vi "Load Outputs.vi"(8 "error in (no error)":errorcluster, 11 "DiscreteRangeControl in":refnum<class "DiscreteRangeControl.lvclass">) -> (0 "error out":errorcluster, 3 "DiscreteRangeControl out":refnum<class "DiscreteRangeControl.lvclass">)   [LabVIEW 2020, in "VolatusControl.lvlib" / "DiscreteRangeControl.lvclass"]
uses:
  DiscreteRangeControl.lvclass
  DiscreteRangeControl.lvclass/DiscreteRangeControl.ctl
  lv-cdm/CDM-Config/Config Element/Config Element.lvclass
  Volatus/MessageQ/MessageQ.lvclass
  Control Action.ctl
  VolatusControl.lvlib
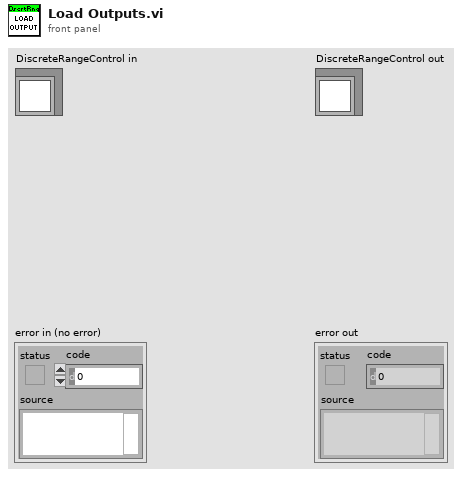
[diagram p1: front panel]
types:
  T1 = typedef "VolatusControl.lvlib/Control Action.ctl" = cluster{"Channel":string, "MsgQ":refnum<class "MessageQ.lvclass">, "Value":bool}
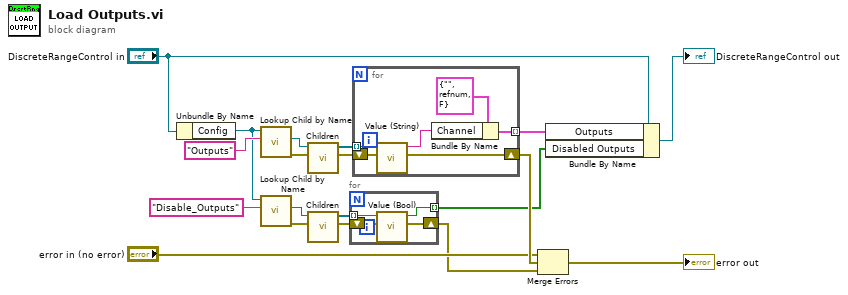
[diagram p0: block diagram]
diagram:
  n1 = Unbundle By Name("DiscreteRangeControl in") -> ("Config"=w9:refnum<class "Config Element.lvclass">)
  n2 = call "Lookup Child by Name.vi"("Name"="Outputs", "Config Element in"=w9) -> ("error out"=w15:errorcluster, "Child"=w14:refnum<class "Config Element.lvclass">)  [unwired: 6 in, 2 out]
  n3 = call "Lookup Child by Name.vi"("Name"="Disable_Outputs", "Config Element in"=w9) -> ("error out"=w6:errorcluster, "Child"=w7:refnum<class "Config Element.lvclass">)  [unwired: 6 in, 2 out]
  n4 = call "Children.vi"("error in (no error)"=w15, "Config Element in"=w14) -> ("error out"=w12:errorcluster, "Elements"=w13:refnum<class "Config Element.lvclass">[])  [unwired: 8 in]
  n5 = call "Children.vi"("error in (no error)"=w6, "Config Element in"=w7) -> ("error out"=w5:errorcluster, "Elements"=w4:refnum<class "Config Element.lvclass">[])  [unwired: 8 in]
  n6 = for {
    shift-right: [w21] -> w1
    shift-left: w5 -> [w23]
    tunnel: w4 -> [w22] mode=indexing
    tunnel: [w20] -> w3 mode=indexing
    n7 = call "Value (Bool).vi"("error in (no error)"=w23, "Config Element in"=w22) -> ("error out"=w21:errorcluster, "Bool Value"=w20:bool)  [unwired: 8 in]
  }
  n8 = for {
    tunnel: w13 -> [w29] mode=indexing
    shift-right: [w24] -> w19
    shift-left: w12 -> [w28]
    tunnel: [w25] -> w10 mode=indexing
    n9 = call "Value (String).vi"("error in (no error)"=w28, "Config Element in"=w29) -> ("error out"=w24:errorcluster, "String Value"=w26:string)  [unwired: 8 in]
    n10 = Bundle By Name(cluster=T1 {"Channel"="", "MsgQ"=refnum, "Value"=FALSE} ("Action"), "Channel"=w26) -> (w25:T1)
  }
  n11 = Merge Errors("error in (no error)", w19, w1) -> (→"error out":errorcluster)
  n12 = Bundle By Name(cluster="DiscreteRangeControl in", "Outputs"=w10, "Disabled Outputs"=w3) -> (→"DiscreteRangeControl out":refnum<class "DiscreteRangeControl.lvclass">)
